vi "GitCount.vi"(8 "error in (no error)":errorcluster, 9 "Directory":path=path "", 11 "Git exec":string="git") -> (0 "error out":errorcluster, 1 "Directory out":path, 2 "Count":u32, 3 "Git exec out":string="git")   [LabVIEW 2013]
uses:
  GitCmd.vi
  <vilib>/dlg_ctls.llb/Space Constant.vi
  GitUtils/PathtoDirPath.vi
  <vilib>/Platform/system.llb/System Exec.vi
  <vilib>/Utility/error.llb/Error Cluster From Error Code.vi
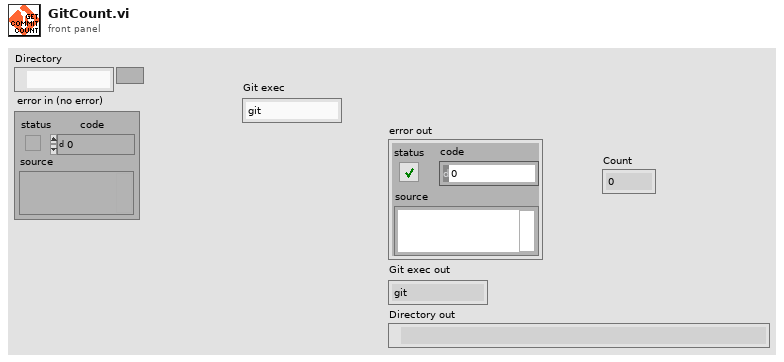
[diagram p1: front panel]
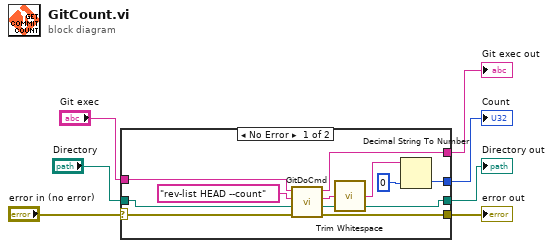
[diagram p0: block diagram]
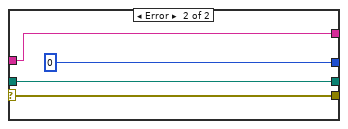
[diagram p2: hidden frame]
diagram:
  n1 = case shown="No Error" "error in (no error)" {
    selector: "error in (no error)" -> [w14 w22]
    tunnel: "Git exec" -> [w11 w20]
    tunnel: "Directory" -> [w13 w21]
    tunnel: [w18 w22] -> w5
    tunnel: [w17 w21] -> w3
    tunnel: [w16 w20] -> w2
    tunnel: [w9 u32 0 ("default (0 I32)")] -> w1
    frame No Error {
      n2 = call "GitDoCmd.vi"("error in (no error)"=w14, "Working Path"=w13, "Git command"="rev-list HEAD --count" ("string"), "Git exec"=w11) -> ("error out"=w18:errorcluster, "Working Path out"=w17:path, "Returned stdout"=w12:string, "Git exec out"=w16:string)  [unwired: 3 in]
      n3 = call <vilib>:"Trim Whitespace.vi"("string"=w12) -> ("trimmed string"=w10:string)  [unwired: 1 in]
      n4 = Decimal String To Number(string=w10, default (0L)=u32 0 ("default (0 I32)")) -> (number=w9:u32)  [unwired: 1 in, 1 out]
    }
    frame Error {
    }
  }
  "error out" <- w5
  "Git exec out" <- w2
  "Directory out" <- w3
  "Count" <- w1
